vi "Write Y_Source.vi"(8 "error in (no error)":errorcluster, 10 "Y_Source":T1, 11 "Y_H in":refnum<class "Y_H.lvclass">) -> (0 "error out":errorcluster, 3 "Y_H out":refnum<class "Y_H.lvclass">)   [LabVIEW 2019, in "Y_H.lvclass"]
uses:
  Y_H.lvclass
  Reg/ctl/Y_source.ctl
  Y_H.lvclass/Y_H.ctl
  Reg/control.lvlib
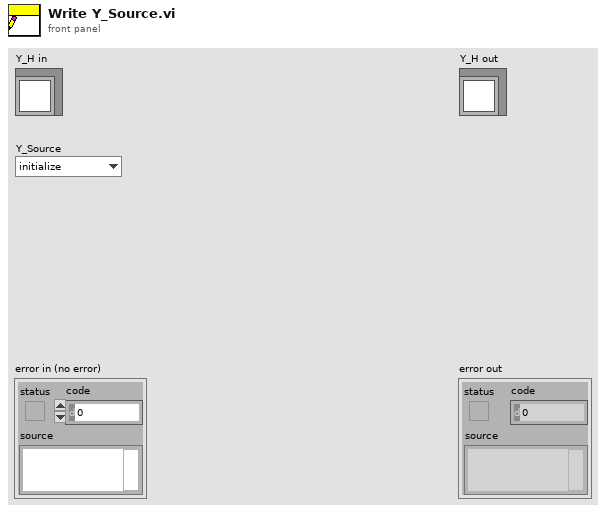
[diagram p1: front panel]
types:
  T1 = typedef "control.lvlib/Y_source.ctl" = enum8{"initialize", "local disabled", "local hand", "hand", "auto", "dist"}
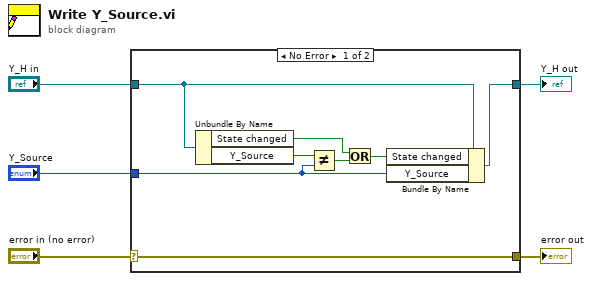
[diagram p0: block diagram]
diagram:
  n1 = case shown="No Error" "error in (no error)" {
    selector: "error in (no error)" -> [w13 w14]
    tunnel: [w13 w14] -> w4
    tunnel: [w12 w15] -> w2
    tunnel: "Y_H in" -> [w11 w15]
    tunnel: "Y_Source" -> [w9 _]
    frame No Error {
      n2 = Unbundle By Name(w11) -> ("State changed"=w6:bool, "Y_Source"=w10:T1)
      n3 = Not Equal?(x=w10, y=w9) -> (x != y?=w7:bool)
      n4 = Or(x=w6, y=w7) -> (x .or. y?=w8:bool)
      n5 = Bundle By Name(cluster=w11, "State changed"=w8, "Y_Source"=w9) -> (w12:refnum<class "Y_H.lvclass">)
    }
    frame Error {
    }
  }
  "error out" <- w4
  "Y_H out" <- w2
